vi "TDC_DAQV19_muon.vi"(8 "error in (no error)":errorcluster, 9 "stop":bool=TRUE, 10 "save data":bool=TRUE, 11 "SMA mode":bool=TRUE) -> (3 "rate":dbl)   [LabVIEW 2017]
uses:
  <vilib>/Utility/file.llb/Write Delimited Spreadsheet (DBL).vi
  <vilib>/Utility/file.llb/Write Delimited Spreadsheet (I64).vi
panel:
  out "substring 2":string
  out "error out 3":errorcluster
  out "substring":string
  in  "factor":i32=128
  in  "displayCR":bool=TRUE
  in  "Counter Setting":dbl=100000.0 format="%#_13g"
  in  "replace dat":bool
  in  "append csv":bool=TRUE
  out "concatenated string":string
  out "number":u32=23
  out "element":string
  out "fine":u64=375 format="%x"
  in  "UDP Config":bool=TRUE
  in  "data  path":path=path "G:/tdc/2017"
  out "cal 2":u64[](graph)
  in  "Thresholds (mV)":u16[](array[numeric])=[580, 580, 580, 580, 600, 600, 600, 600, 580, 580, 600, 600, 600, 600, 600, 600, 580, 580, 600, 600, 600, 600, 600, 600, 580, 580, 600, 600, 600, 600, 600, 600]
  out "error out 2":errorcluster={"status"=TRUE, "code"=1, "source"="Dequeue Element in TDC_DAQV18_NewStructure.vi"}
  in  "display":bool=TRUE
  in  "Thresholds":u16=580
  in  "one key for threshold":bool=TRUE
  in  "RST":bool
  in  "通道数量":i32=64
  out "Cal Table":u32[](array[numeric])
  in  "channel for cal":i32
  out "channel number":u64
  in  "bytes to read":i32=320
  out "Calibration Counter":i32=100000
  out "Event index":i32=97959
  out "cal":u32[](graph)
  out "error out":errorcluster
  out "appended path":path=path "G:/tdc/2017/test_20240612_084516.dat"
  in  "filename":string="test"
  in  "Events":i32=110000 min=1
  in  "timeout (ms)":i32=10000
  in  "address":string="192.168.10.23"
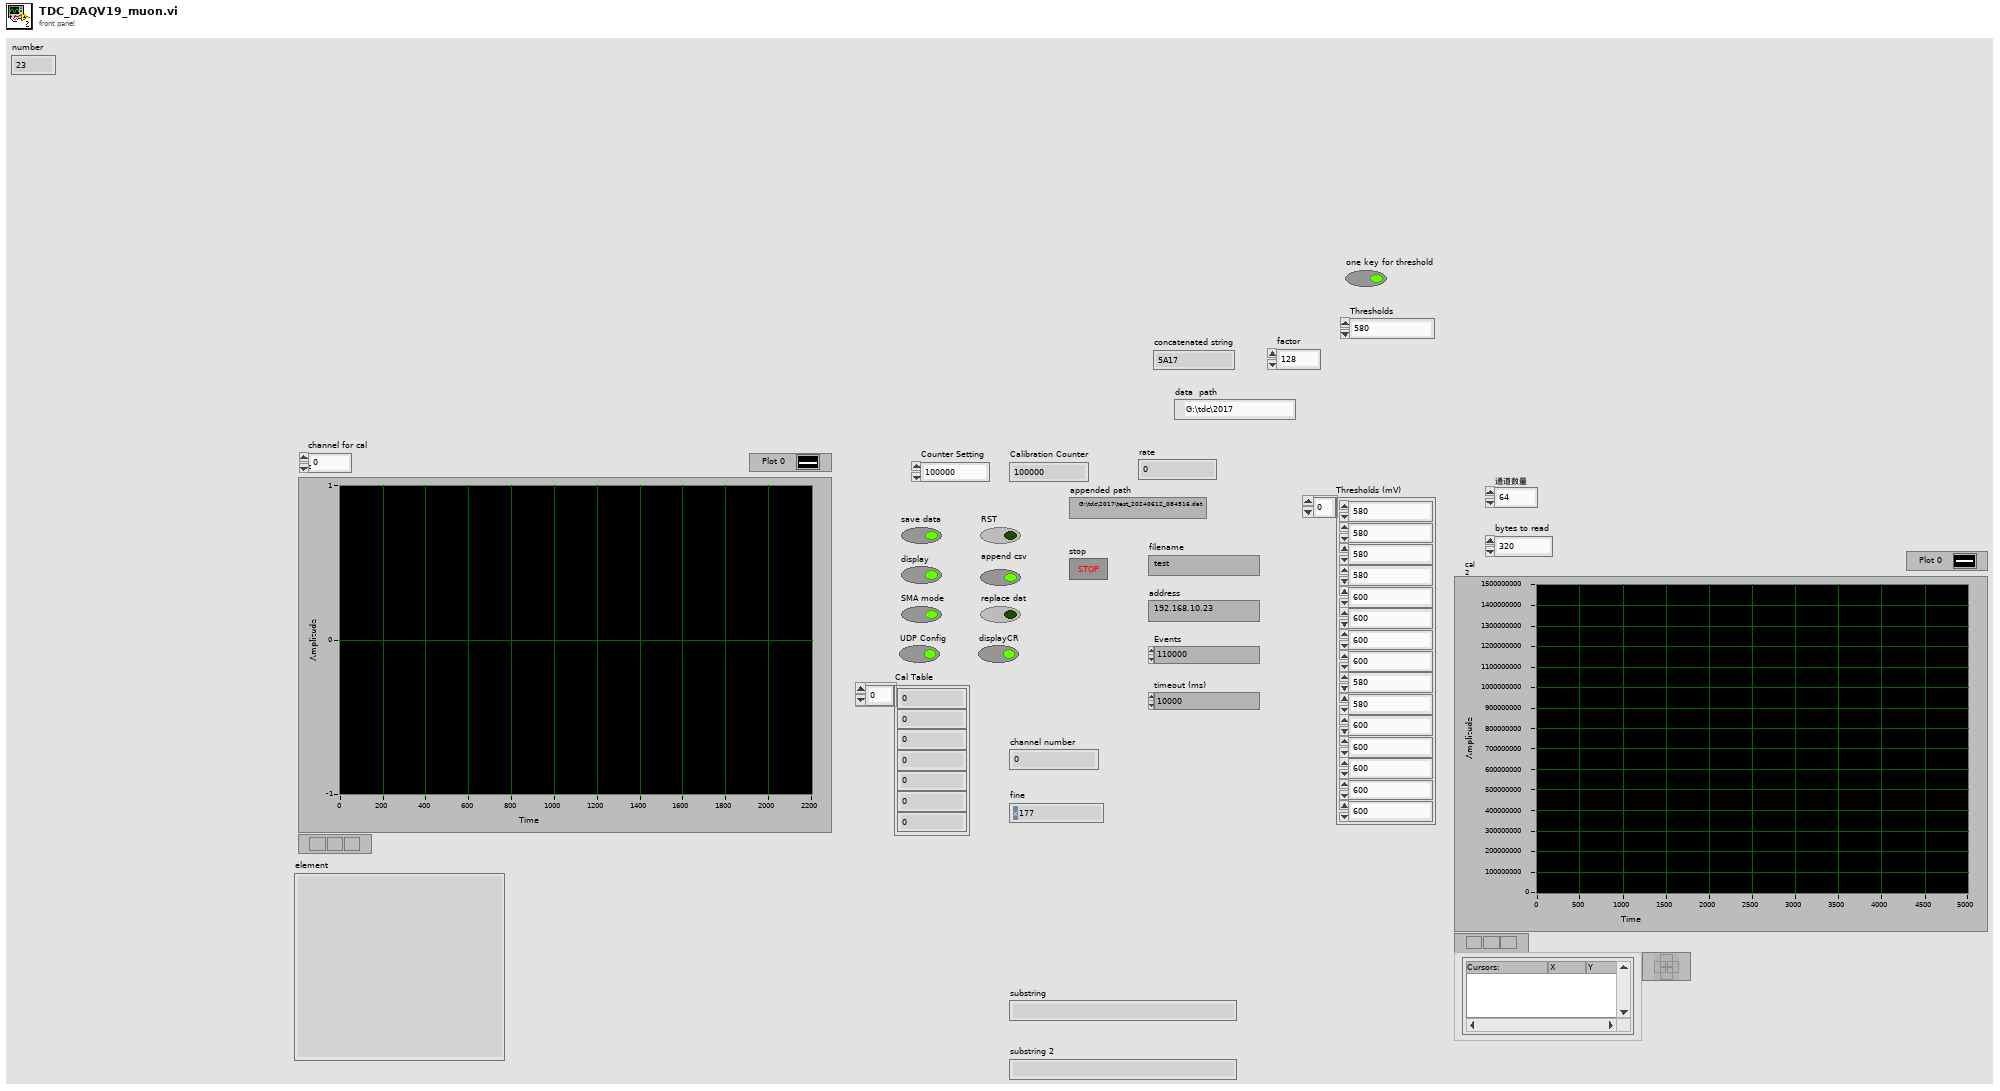
[diagram p1: front panel]
types:
  T1 = enum16{"open", "replace", "create", "open or create", "replace or create", "replace or create with confirmation"}
  T2 = enum16{"Standard", "Buffered", "CRLF", "Immediate"}
  T3 = enum16{"big-endian, network order", "native, host order", "little-endian"}
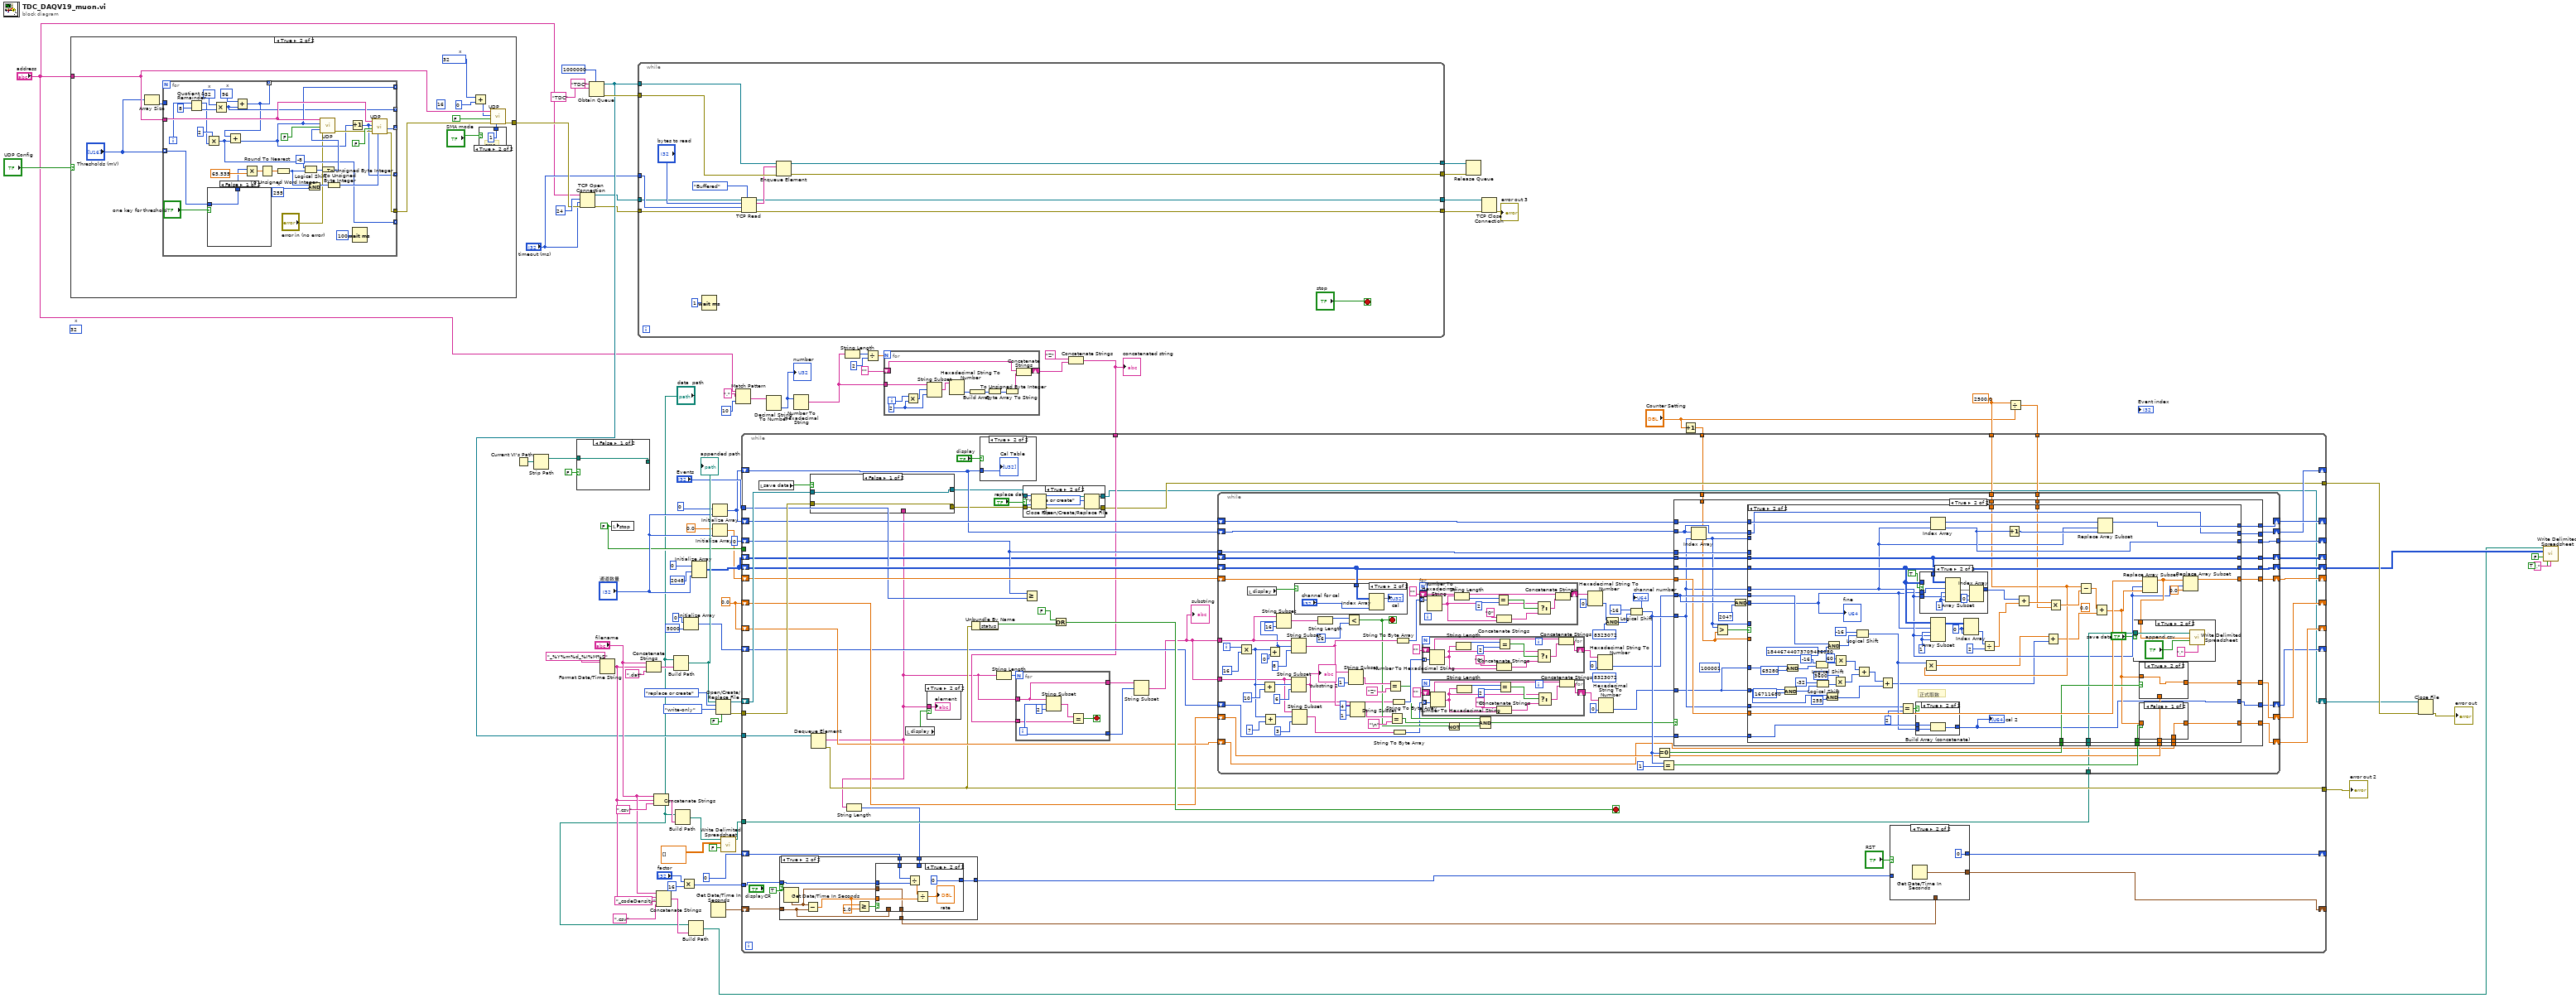
[diagram p0: block diagram]
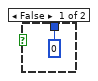
[diagram p3: hidden frame]
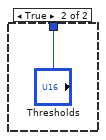
[diagram p4: hidden frame]
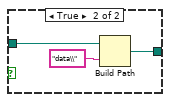
[diagram p5: hidden frame]
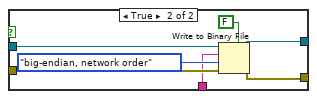
[diagram p7: hidden frame]
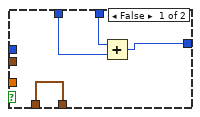
[diagram p10: hidden frame]
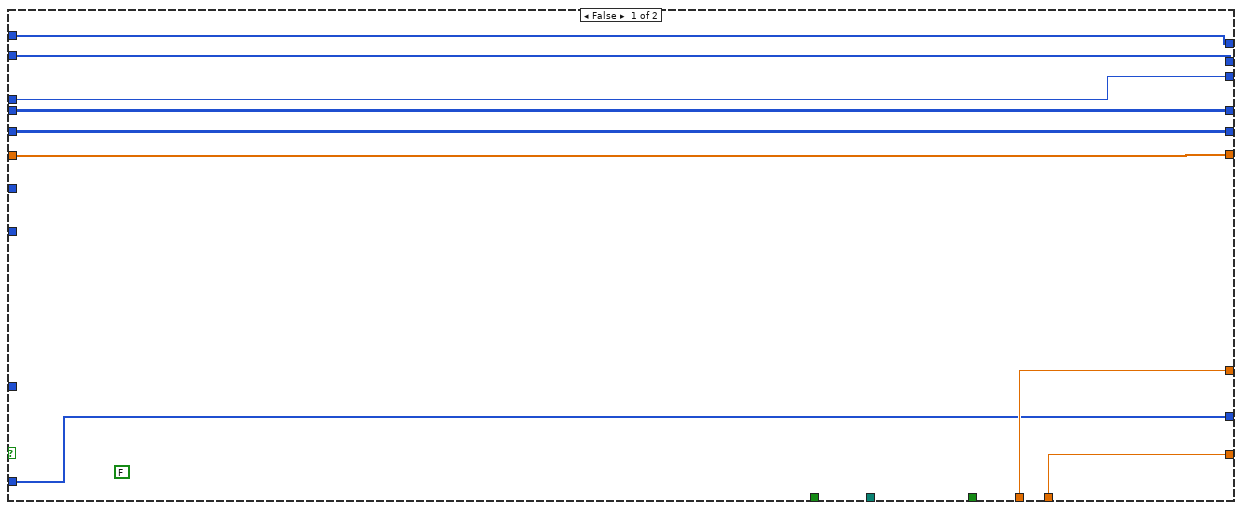
[diagram p14: hidden frame]
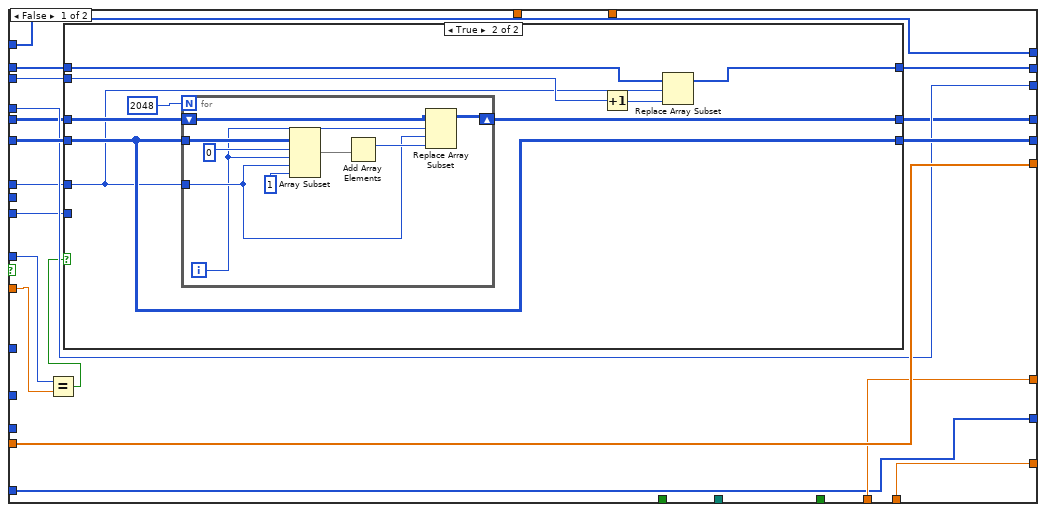
[diagram p15: hidden frame]
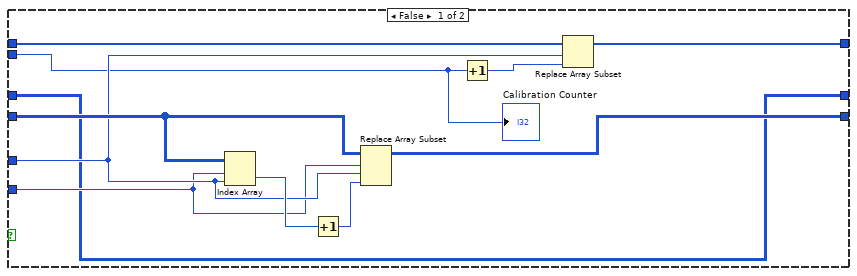
[diagram p16: hidden frame]
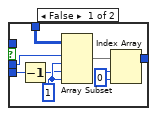
[diagram p19: hidden frame]
diagram:
  w10 = 2500.0 ("x")
  (unwired) u16 32  # x
  w54 = FALSE ("stop")
  w64 = 0.0
  n1 = case shown="True" "UDP Config" {
    tunnel: "address" -> [_ w97]
    tunnel: [_ w94] -> w55
    frame False {
    }
    frame True {
      (unwired) u32 16 ("Address")
      w88 = u16 32  # x
      n2 = Array Size(array="Thresholds (mV)") -> (size(s)=w91:i32)
      n3 = for {
        tunnel: w97 -> [w127]
        tunnel: "Thresholds (mV)" -> [w113] mode=indexing
        tunnel: [w121] -> _ mode=indexing
        tunnel: [w116] -> w95
        tunnel: w91 -> [_]
        tunnel: [w107] -> _ mode=indexing
        tunnel: [w106] -> _ mode=indexing
        tunnel: [w105] -> _ mode=indexing
        tunnel: [w104] -> _ mode=indexing
        tunnel: [w103] -> _ mode=indexing
        i -> [w108]
        w109 = u16 96  # x
        w110 = u16 32  # x
        w123 = u16 255  # x
        n4 = Quotient & Remainder(x=w108, y=8) -> (x-y*floor(x/y)=w102:i32, floor(x/y)=w111:i32)
        n5 = Multiply(x=2, y=w102) -> (x*y=w103:i32)
        n6 = case shown="False" "one key for threshold" {
          tunnel: [w133 "Thresholds"] -> w114
          tunnel: w113 -> [w133 _]
          frame False {
          }
          frame True {
          }
        }
        n7 = Multiply(x=w110, y=w111) -> (x*y=w105:i32)
        n8 = Add(x=w109, y=w105) -> (x+y=w104:i32)
        n9 = Add(x=w104, y=w103) -> (x+y=w107:i32)
        n10 = Multiply(x=w114, y=65.535) -> (x*y=w130:dbl)
        n11 = Round To Nearest(number=w130) -> (nearest integer value=w128:dbl)
        n12 = To Unsigned Word Integer(number=w128) -> (unsigned 16bit integer=w118:u16)
        n13 = Logical Shift(y=i16 -8, x=w118) -> (x << y=w125:u16)
        n14 = And(x=w118, y=w123) -> (x .and. y?=w122:u16)
        n15 = To Unsigned Byte Integer(number=w125) -> (unsigned 8bit integer=w124:u8)
        n16 = call "UDP.vi"("In"=w124, "error in (no error)"="error in (no error)", "Read (TRUE)"=FALSE, "Address"=w107, "IP address"=w127) -> ("error out"=w117:errorcluster)  [unwired: 4 in, 1 out]
        n17 = To Unsigned Byte Integer(number=w122) -> (unsigned 8bit integer=w120:u8)
        n18 = Increment(x=w107) -> (x+1=w106:i32)
        n19 = Wait (ms)(milliseconds to wait=u32 100) -> ()  [unwired: 1 out]
        n20 = call "UDP.vi"("In"=w120, "error in (no error)"=w117, "Read (TRUE)"=FALSE, "Address"=w106, "IP address"=w127) -> ("error out"=w116:errorcluster, "Out"=w121:u8)  [unwired: 4 in]
      }
      n21 = Add(x=w88, y=u32 0 ("Address")) -> (x+y=w87:u32)
      n22 = case shown="True" "SMA mode" {
        tunnel: [u8 0 ("In") u8 1 ("In")] -> w93
        frame False {
        }
        frame True {
          # "sma"
        }
      }
      n23 = call "UDP.vi"("In"=w93, "error in (no error)"=w95, "Read (TRUE)"=FALSE, "Address"=w87, "IP address"=w97) -> ("error out"=w94:errorcluster)  [unwired: 4 in, 1 out]
    }
  }
  n24 = Current VI's Path() -> (path=w80:path)
  n25 = Strip Path(path=w80) -> (stripped path=w79:path)  [unwired: 1 out]
  n26 = case shown="False" FALSE {
    tunnel: w79 -> [w135 w137]
    tunnel: [w135 w136] -> _
    frame False {
    }
    frame True {
      n27 = Build Path(base path=w137, name or relative path="data\\") -> (appended path=w136:path)
    }
  }
  n28 = TCP Open Connection(address="address", remote port or service name=u16 24 ("port"), timeout ms (60000)="timeout (ms)", error in (no error)=w55) -> (connection ID=w38:refnum<k5>, error out=w39:errorcluster)  [unwired: 1 in]
  n29 = Obtain Queue(max queue size (-1, unlimited)=1000000, name (unnamed)="TDC", element data type="TDC" ("name (unnamed)")) -> (queue out=w40:refnum<queue>, error out=w41:errorcluster)  [unwired: 2 in, 1 out]
  n30 = Format Date/Time String(time format string (%c)="_%Y%m%d_%I%M%S") -> (date/time string=w52:string)  [unwired: 2 in]
  n31 = local write "stop"(w54) -> ()
  n32 = while {
    tunnel: w40 -> [w152]
    tunnel: w41 -> [w151]
    tunnel: w39 -> [w149]
    tunnel: "timeout (ms)" -> [w148]
    tunnel: w38 -> [w147]
    tunnel: [w145] -> w37
    tunnel: [w144] -> w36
    tunnel: [w142] -> w35
    tunnel: [w141] -> w34
    stop <- "stop" stop-if-true
    n33 = Wait (ms)(milliseconds to wait=u32 1) -> ()  [unwired: 1 out]
    n34 = TCP Read(connection ID=w147, bytes to read="bytes to read", error in (no error)=w149, 7:T2."Buffered" ("mode (standard)"), 9:w148) -> (connection ID out=w145:refnum<k5>, data out=w146:string, error out=w144:errorcluster)
    n35 = Enqueue Element(queue=w152, element=w146, error in (no error)=w151) -> (queue out=w142:refnum<queue>, error out=w141:errorcluster)  [unwired: 1 in, 1 out]
  }
  n36 = Concatenate Strings("filename", w52, ".dat") -> (w78:string)
  n37 = Concatenate Strings("filename", w52, ".csv") -> (w66:string)
  n38 = Concatenate Strings("filename", w52, "_codeDensity" ("string"), ".csv") -> (w49:string)
  n39 = Build Path(base path="data  path", name or relative path=w78) -> (appended path=w77:path)
  "appended path" <- w77
  n40 = Build Path(base path="data  path", name or relative path=w66) -> (appended path=w61:path)
  n41 = Multiply(x="factor", y=16) -> (x*y=w3:i32)
  n42 = Initialize Array(u32 0 ("element"), 5000 ("dimension size")) -> (w28:u32[])
  n43 = Build Path(base path="data  path", name or relative path=w49) -> (appended path=w46:path)
  n44 = Initialize Array(u32 0 ("element"), 2048 ("dimension size"), "通道数量") -> (w63:u32[][])
  n45 = Get Date/Time In Seconds() -> (seconds since 1Jan1904=w56:timestamp)
  n46 = Initialize Array(u32 0 ("element"), "通道数量") -> (w65:u32[])
  n47 = Initialize Array(0.0, "通道数量") -> (w30:dbl[])
  n48 = Open/Create/Replace File(file path (use dialog)=w77, operation (0:open)=T1."replace or create", access (0:read/write)=enum16{"read/write", "read-only", "write-only"}."write-only", disable buffering (F)=FALSE) -> (refnum out=w82:refnum<file>, error out=w81:errorcluster)  [unwired: 2 in, 1 out]
  n49 = call-poly <vilib>:"Write Delimited Spreadsheet.vi"("file path (dialog if empty)"=w61, "2D data"=dbl[][] [], "append to file? (new file:F)"=FALSE) -> ("new file path (Not A Path if cancelled)"=w60:path)  [unwired: 11 in, 1 out]
  n50 = Match Pattern(string="address", regular expression="." ("search string"), offset (0)=10) -> (after substring=w17:string)  [unwired: 3 out]
  n51 = Decimal String To Number(string=w17) -> (number=w16:i32)  [unwired: 2 in, 1 out]
  "number" <- w16
  n52 = Number To Hexadecimal String(2:w16) -> (0:w14:string)  [unwired: 1 in]
  n53 = String Length(string=w14) -> (length=w22:i32)
  n54 = Divide(x=w22, y=2) -> (x/y=w23:dbl)
  n55 = for {
    N: w23 -> [_]
    shift-right: [w163] -> w13
    shift-left: "" ("format string") -> [w162]
    tunnel: w14 -> [w153]
    i -> [w161]
    w155 = 2 ("y")
    n56 = Multiply(x=w161, y=w155) -> (x*y=w154:i32)
    n57 = String Subset(string=w153, offset (0)=w154, length (rest)=w155) -> (substring=w156:string)
    n58 = Hexadecimal String To Number(string=w156) -> (number=w160:u32)  [unwired: 2 in, 1 out]
    n59 = Build Array(w160) -> (w159:u32[])
    n60 = To Unsigned Byte Integer(number=w159) -> (unsigned 8bit integer=w158:u8[])
    n61 = Byte Array To String(unsigned byte array=w158) -> (string=w157:string)
    n62 = Concatenate Strings(w162, w157) -> (w163:string)
  }
  n63 = Concatenate Strings("Z", w13) -> (w12:string)
  "concatenated string" <- w12
  n64 = Release Queue(queue=w35, error in (no error)=w34) -> ()  [unwired: 1 in, 3 out]
  n65 = TCP Close Connection(connection ID=w37, error in (no error)=w36) -> (error out=→"error out 3":errorcluster)  [unwired: 1 in, 1 out]
  n66 = Increment(x="Counter Setting") -> (x+1=w6:dbl)
  n67 = Divide(x=w10, y="Counter Setting") -> (x/y=w9:dbl)
  n68 = while {
    tunnel: w81 -> [w217]
    tunnel: [w191] -> w33
    tunnel: [w175] -> w74
    shift-right: [w214] -> w47
    shift-left: w63 -> [w215]
    shift-right: [w200] -> _
    shift-left: w30 -> [w213]
    tunnel: "Events" -> [w211]
    shift-right: [w210] -> _
    shift-left: w65 -> [w209]
    shift-right: [w208] -> _
    shift-left: u32 0 ("element") -> [w207]
    shift-right: [w206] -> _
    shift-left: w65 -> [w193]
    shift-right: [w205] -> _
    shift-left: w64 -> [w202]
    shift-right: [w204] -> _
    shift-left: w64 -> [w203]
    shift-right: [w195] -> _
    shift-left: w63 -> [w201]
    tunnel: w60 -> [w187]
    shift-right: [w199] -> _
    shift-left: 0 -> [w169]
    shift-right: [w197] -> _
    shift-left: w56 -> [w196]
    tunnel: w54 -> [_]
    tunnel: w40 -> [w192]
    shift-right: [w188] -> _
    shift-left: w28 -> [w189]
    tunnel: w12 -> [w183]
    tunnel: w10 -> [w181]
    tunnel: w9 -> [w180]
    shift-right: [w174] -> w8
    shift-left: w82 -> [w216]
    tunnel: w6 -> [w173]
    tunnel: w3 -> [w166]
    stop <- w212 stop-if-true
    n69 = local read "save data"() -> (w168:bool)
    n70 = Dequeue Element(queue=w192) -> (element=w179:string, error out=w191:errorcluster)  [unwired: 2 in, 2 out]
    n71 = case shown="False" w168 {
      tunnel: w217 -> [w219 w227]
      tunnel: w216 -> [w220 w226]
      tunnel: w179 -> [_ w223]
      tunnel: [w220 w222] -> w178
      tunnel: [w219 w221] -> w176
      frame False {
      }
      frame True {
        n72 = Write to Binary File(file (use dialog)=w226, data=w223, error in=w227, 5:FALSE ("prepend array or string size? (T)"), 9:T3."big-endian, network order" ("byte order (0:big-endian, network order)")) -> (refnum out=w222:refnum<file>, error out=w221:errorcluster)  [unwired: 1 in, 1 out]
      }
    }
    n73 = String Length(string=w179) -> (length=w170:i32)
    n74 = case shown="True" TRUE {
      tunnel: w196 -> [w244 w249]
      tunnel: [w244 w250] -> w172
      tunnel: w169 -> [w243 w248]
      tunnel: w170 -> [_ w247]
      tunnel: [w243 w246] -> w171
      tunnel: w166 -> [_ w245]
      frame False {
      }
      frame True {
        n75 = Get Date/Time In Seconds() -> (seconds since 1Jan1904=w251:timestamp)
        n76 = Subtract(x=w251, y=w249) -> (x-y=w253:dbl)
        n77 = Greater Or Equal?(x=w253, y=1.0) -> (x >= y?=w254:bool)
        n78 = case shown="True" w254 {
          tunnel: w253 -> [_ w265]
          tunnel: w251 -> [_ w263]
          tunnel: [w258 w263] -> w250
          tunnel: w249 -> [w258 _]
          tunnel: w248 -> [w257 w260]
          tunnel: w247 -> [w256 _]
          tunnel: [w255 0] -> w246
          tunnel: w245 -> [_ w259]
          frame False {
            n79 = Add(x=w256, y=w257) -> (x+y=w255:i32)
          }
          frame True {
            n80 = Divide(x=w260, y=w259) -> (x/y=w262:dbl)
            n81 = Divide(x=w262, y=w265) -> (x/y=→"rate":dbl)
          }
        }
      }
    }
    n82 = local read "display"() -> (w167:bool)
    n83 = case shown="True" w167 {
      tunnel: w179 -> [_ w218]
      frame False {
      }
      frame True {
        "element" <- w218
      }
    }
    n84 = Unbundle By Name(w191) -> ("status"=w190:bool)
    n85 = case shown="True" "display" {
      tunnel: w193 -> [_ w266]
      frame False {
      }
      frame True {
        "Cal Table" <- w266
      }
    }
    n86 = String Length(string=w179) -> (length=w186:i32)
    n87 = for {
      N: w186 -> [_]
      tunnel: w179 -> [w239]
      tunnel: [w239] -> w185
      tunnel: [w238] -> w184
      tunnel: w183 -> [w237]
      i -> [w238]
      stop <- w240 stop-if-true
      n88 = String Subset(string=w239, offset (0)=w238, length (rest)=2 ("length (rest)")) -> (substring=w241:string)
      n89 = Equal?(x=w241, y=w237) -> (x = y?=w240:bool)
    }
    n90 = case shown="True" "replace dat" {
      tunnel: w178 -> [w229 w235]
      tunnel: [w229 w234] -> w174
      tunnel: w176 -> [w228 w231]
      tunnel: [w228 w230] -> w175
      frame False {
      }
      frame True {
        n91 = Close File(refnum=w235, error in=w231) -> (path=w236:path, error out=w232:errorcluster)
        n92 = Open/Create/Replace File(file path (use dialog)=w236, error in=w232, operation (0:open)=T1."replace or create") -> (refnum out=w234:refnum<file>, error out=w230:errorcluster)  [unwired: 3 in, 1 out]
      }
    }
    n93 = Greater Or Equal?(x=w207, y=w211) -> ()  [unwired: 1 out]
    n94 = Or(x=FALSE, y=w190) -> (x .or. y?=w212:bool)
    n95 = String Subset(string=w185, offset (0)=w184) -> (substring=w164:string)  [unwired: 1 in]
    "substring" <- w164
    n96 = while {
      tunnel: w164 -> [w291]
      shift-right: [w344] -> w214
      shift-left: w215 -> [w342]
      shift-right: [w340] -> w200
      shift-left: w213 -> [w341]
      shift-right: [w335] -> w210
      shift-left: w209 -> [w334]
      tunnel: [w333] -> w208
      tunnel: w207 -> [w332]
      shift-right: [w330] -> w206
      shift-left: w193 -> [w331]
      shift-right: [w325] -> w205
      shift-left: w202 -> [w323]
      shift-right: [w321] -> w204
      shift-left: w203 -> [w322]
      tunnel: w187 -> [w320]
      shift-right: [w319] -> w195
      shift-left: w201 -> [w285]
      shift-right: [w316] -> w188
      shift-left: w189 -> [w317]
      tunnel: w164 -> [w277]
      tunnel: w181 -> [w293]
      tunnel: w180 -> [w292]
      tunnel: w173 -> [w284]
      i -> [w345]
      stop <- w287 stop-if-true
      (unwired) u64 8323072 ("port")
      n97 = Multiply(x=w345, y=16 ("length (rest)")) -> (x*y=w278:i32)
      n98 = local read "display"() -> (w318:bool)
      n99 = Add(x=w278, y=10 ("length (rest)")) -> (x+y=w308:i32)
      n100 = Add(x=w278, y=7 ("length (rest)")) -> (x+y=w280:i32)
      n101 = Add(x=w278, y=0 ("length (rest)")) -> (x+y=w290:i32)
      n102 = String Subset(string=w291, offset (0)=w290, length (rest)=16 ("y")) -> (substring=w288:string)
      n103 = String Subset(string=w291, offset (0)=w290, length (rest)=8 ("length (rest)")) -> (substring=w294:string)
      n104 = String Subset(string=w277, offset (0)=w308, length (rest)=6 ("length (rest)")) -> (substring=w283:string)
      "substring 2" <- w283
      n105 = String Subset(string=w277, offset (0)=w280, length (rest)=3 ("length (rest)")) -> (substring=w273:string)
      n106 = case shown="True" w318 {
        tunnel: w342 -> [_ w371]
        frame False {
        }
        frame True {
          n107 = Index Array(array=w371, index (col)="channel for cal") -> (element=→"cal":u32[])  [unwired: 1 in]
        }
      }
      n108 = String Length(string=w288) -> (length=w339:i32)
      n109 = Less?(x=w339, y=16) -> (x < y?=w287:bool)
      n110 = String Subset(string=w294, length (rest)=1 ("length (rest)")) -> (substring=w313:string)  [unwired: 1 in]
      n111 = String Subset(string=w294, offset (0)=4, length (rest)=1 ("length (rest)")) -> (substring=w295:string)
      n112 = Equal?(x=w313, y="Z" ("format string")) -> (x = y?=w297:bool)
      n113 = Equal?(x=w295, y="\n" ("format string")) -> (x = y?=w296:bool)
      n114 = String To Byte Array(string=w283) -> (unsigned byte array=w305:u8[])
      n115 = String To Byte Array(string=w273) -> (unsigned byte array=w272:u8[])
      n116 = String To Byte Array(string=w294) -> (unsigned byte array=w347:u8[])
      n117 = for {
        shift-right: [w559] -> w302
        shift-left: "" ("format string") -> [w556]
        tunnel: w347 -> [w560] mode=indexing
        n118 = Number To Hexadecimal String(2:w560) -> (0:w552:string)  [unwired: 1 in]
        n119 = String Length(string=w552) -> (length=w558:i32)
        n120 = Equal?(x=w558, y=2) -> (x = y?=w555:bool)
        n121 = Concatenate Strings("0" ("format string"), w552) -> (w554:string)
        n122 = Select(t=w552, s=w555, f=w554) -> (s? t:f=w551:string)
        n123 = Concatenate Strings(w556, w551) -> (w559:string)
      }
      n124 = for {
        shift-right: [w367] -> w303
        shift-left: "" ("format string") -> [w359]
        tunnel: w305 -> [w368] mode=indexing
        n125 = Number To Hexadecimal String(2:w368) -> (0:w361:string)  [unwired: 1 in]
        n126 = String Length(string=w361) -> (length=w366:i32)
        n127 = Concatenate Strings("0" ("format string"), w361) -> (w363:string)
        n128 = Equal?(x=w366, y=2) -> (x = y?=w364:bool)
        n129 = Select(t=w361, s=w364, f=w363) -> (s? t:f=w360:string)
        n130 = Concatenate Strings(w359, w360) -> (w367:string)
      }
      n131 = for {
        shift-right: [w357] -> w276
        shift-left: "" ("format string") -> [w349]
        tunnel: w272 -> [w358] mode=indexing
        n132 = Number To Hexadecimal String(2:w358) -> (0:w351:string)  [unwired: 1 in]
        n133 = String Length(string=w351) -> (length=w356:i32)
        n134 = Concatenate Strings("0" ("format string"), w351) -> (w353:string)
        n135 = Equal?(x=w356, y=2) -> (x = y?=w354:bool)
        n136 = Select(t=w351, s=w354, f=w353) -> (s? t:f=w350:string)
        n137 = Concatenate Strings(w349, w350) -> (w357:string)
      }
      n138 = Not(x=w287) -> (.not. x?=w286:bool)
      n139 = Compound Arithmetic op=AND(w297, w296, w286) -> (w311:bool)
      n140 = Hexadecimal String To Number(string=w302, default (0uL)=u64 0 ("default (0 U32)")) -> (number=w343:u64)  [unwired: 1 in, 1 out]
      n141 = Hexadecimal String To Number(string=w303, default (0uL)=u64 0 ("default (0 U32)")) -> (number=w301:u64)  [unwired: 1 in, 1 out]
      n142 = Hexadecimal String To Number(string=w276, default (0uL)=u64 0 ("default (0 U32)")) -> (number=w271:u64)  [unwired: 1 in, 1 out]
      n143 = And(x=w343, y=u64 8323072 ("port")) -> (x .and. y?=w336:u64)
      n144 = Logical Shift(y=i16 -16, x=w336) -> (x << y=w328:u64)
      "channel number" <- w328
      n145 = Equal To 0?(x=w328) -> (x = 0?=w326:bool)
      n146 = Equal?(x=w328, y=u64 1) -> (x = y?=w324:bool)
      n147 = case shown="True" w311 {
        tunnel: w301 -> [_ w411]
        tunnel: w332 -> [w377 w401]
        tunnel: w342 -> [w380 w410]
        tunnel: [w380 w409] -> w344
        tunnel: [w379 w406] -> w340
        tunnel: w341 -> [w379 w405]
        tunnel: w328 -> [_ w385]
        tunnel: w334 -> [w378 w404]
        tunnel: [w378 w403] -> w335
        tunnel: [w377 w402] -> w333
        tunnel: w331 -> [w376 w400]
        tunnel: [w376 w399] -> w330
        tunnel: w326 -> [_ w398]
        tunnel: w323 -> [w375 w397]
        tunnel: [w375 w396] -> w325
        tunnel: w324 -> [_ w395]
        tunnel: w322 -> [w374 w394]
        tunnel: [w374 w393] -> w321
        tunnel: w285 -> [w373 w391]
        tunnel: [w373 w390] -> w319
        tunnel: w320 -> [_ w389]
        tunnel: w317 -> [w372 w387]
        tunnel: [w372 w386] -> w316
        tunnel: w293 -> [_ w384]
        tunnel: w292 -> [_ w383]
        tunnel: w284 -> [_ w382]
        tunnel: w271 -> [_ w381]
        frame False {
          (unwired) FALSE
        }
        frame True {
          (unwired) 100001 ("y")
          n148 = Index Array(array=w400, index=w385) -> (element=w392:u32)
          n149 = Greater?(x=w392, y=w382) -> (0:w388:bool)
          n150 = And(x=w411, y=u64 2047 ("port")) -> (x .and. y?=w407:u64)
          n151 = case shown="True" w388 {
            tunnel: w411 -> [_ w523]
            tunnel: w410 -> [w429 w509]
            tunnel: [w428 w509] -> w409
            tunnel: w407 -> [w420 w482]
            tunnel: [w427 w493] -> w406
            tunnel: w405 -> [w427 w516]
            tunnel: w401 -> [w425 _]
            tunnel: w385 -> [w423 w491]
            tunnel: w404 -> [w426 w515]
            tunnel: [w426 w514] -> w403
            tunnel: [w425 w512] -> w402
            tunnel: w392 -> [w421 _]
            tunnel: w400 -> [w424 w511]
            tunnel: [w422 w511] -> w399
            tunnel: w398 -> [_ w504]
            tunnel: w397 -> [w419 w503]
            tunnel: [w419 w502] -> w396
            tunnel: w395 -> [_ w501]
            tunnel: w394 -> [w418 w500]
            tunnel: [w418 w499] -> w393
            tunnel: w392 -> [w416 _]
            tunnel: w382 -> [w413 _]
            tunnel: w391 -> [w415 w495]
            tunnel: [w414 w495] -> w390
            tunnel: w389 -> [_ w494]
            tunnel: w387 -> [w412 w488]
            tunnel: [w412 w486] -> w386
            tunnel: w385 -> [_ w483]
            tunnel: w384 -> [_ w480]
            tunnel: w383 -> [_ w481]
            tunnel: w381 -> [_ w475]
            tunnel: w381 -> [_ w463]
            frame False {
              n152 = Equal?(x=w416, y=w413) -> (x = y?=w417:bool)
              n153 = case shown="True" w417 {
                tunnel: w429 -> [w440 w446]
                tunnel: [w438 w446] -> w428
                tunnel: w424 -> [w436 w444]
                tunnel: w423 -> [w435 w441]
                tunnel: [w433 w443] -> w422
                tunnel: w421 -> [w432 w442]
                tunnel: w420 -> [w431 _]
                tunnel: w415 -> [w430 w448]
                tunnel: [w430 w447] -> w414
                frame False {
                  n154 = Index Array(array=w440, index (row)=w431, index (col)=w435) -> (element=w439:u32)
                  n155 = Increment(x=w439) -> (x+1=w437:u32)
                  n156 = Replace Array Subset(array=w440, new element=w437, index (row)=w431, index (col)=w435) -> (w438:u32[][])
                  n157 = Increment(x=w432) -> (x+1=w434:u32)
                  n158 = Replace Array Subset(array=w436, new element=w434, index=w435) -> (w433:u32[])
                  "Calibration Counter" <- w432
                }
                frame True {
                  n159 = for {
                    N: 2048 -> [_]
                    tunnel: w446 -> [w458]
                    tunnel: w441 -> [w451]
                    shift-right: [w453] -> w447
                    shift-left: w448 -> [w454]
                    i -> [w450]
                    n160 = Array Subset(array=w458, index (row)=0 ("索引"), length (row)=w450, index (col)=w451, length (col)=1 ("长度")) -> (w455:u32[][])
                    n161 = Add Array Elements(numeric array=w455) -> (sum=w452:u32)
                    n162 = Replace Array Subset(array=w454, new element=w452, index (row)=w450, index (col)=w451) -> (w453:u32[][])
                  }
                  n163 = Increment(x=w442) -> (x+1=w445:u32)
                  n164 = Replace Array Subset(array=w444, new element=w445, index=w441) -> (w443:u32[])
                }
              }
            }
            frame True {
              (unwired) 0.0 ("x")
              w506 = 0 ("索引 (行)")
              w508 = 1 ("长度")
              # "正式取数"
              n165 = And(x=w463, y=u64 16711680 ("port")) -> (x .and. y?=w472:u64)
              n166 = And(x=w475, y=u64 65280 ("port")) -> (x .and. y?=w478:u64)
              n167 = Logical Shift(y=i16 -16, x=w478) -> (x << y=w469:u64)
              n168 = Logical Shift(y=i16 -32, x=w472) -> (x << y=w471:u64)
              n169 = And(x=w463, y=u64 255 ("port")) -> (x .and. y?=w462:u64)
              n170 = And(x=w523, y=u64 18446744073709486080 ("port")) -> (x .and. y?=w520:u64)
              n171 = Multiply(x=u64 3600, y=w471) -> (x*y=w466:u64)
              n172 = Multiply(x=u64 60, y=w469) -> (x*y=w467:u64)
              n173 = Logical Shift(y=i16 -16, x=w520) -> (x << y=w487:u64)
              n174 = Add(x=w467, y=w466) -> (x+y=w465:u64)
              n175 = Add(x=w465, y=w462) -> (x+y=w459:u64)
              n176 = Equal?(x=w483, y=u32 2) -> (x = y?=w485:bool)
              n177 = case shown="True" w485 {
                tunnel: w488 -> [w524 w527]
                tunnel: w487 -> [_ w526]
                tunnel: [w524 w525] -> w486
                frame False {
                }
                frame True {
                  n178 = Build Array (concatenate)(w527, w526) -> (w525:u64[])
                }
              }
              "cal 2" <- w486
              n179 = case shown="True" TRUE {
                tunnel: [w534 w542] -> w518
                tunnel: w509 -> [_ _]
                tunnel: w491 -> [w539 w540]
                tunnel: w482 -> [w537 w545]
                tunnel: w495 -> [w538 w546]
                frame False {
                  w533 = 0 ("index (row)")
                  w536 = 1 ("长度")
                  n180 = Decrement(x=w539) -> (x-1=w532:u64)
                  n181 = Array Subset(array=w538, index (row)=w537, length (row)=w536, index (col)=w532, length (col)=w536) -> (w535:u32[][])
                  n182 = Index Array(array=w535, index (row)=w533, index (col)=w533) -> (element=w534:u32)
                }
                frame True {
                  w541 = 0 ("index (row)")
                  w544 = 1 ("长度")
                  n183 = Array Subset(array=w546, index (row)=w545, length (row)=w544, index (col)=w540, length (col)=w544) -> (w543:u32[][])
                  n184 = Index Array(array=w543, index (row)=w541, index (col)=w541) -> (element=w542:u32)
                }
              }
              n185 = Multiply(x=w487, y=w480) -> (x*y=w461:dbl)
              n186 = Index Array(array=w515, index=w491) -> (element=w512:u32)
              n187 = Array Subset(array=w509, index (row)=w482, length (row)=w508, index (col)=w491, length (col)=w508) -> (w507:u32[][])
              n188 = Index Array(array=w507, index (row)=w506, index (col)=w506) -> (element=w505:u32)
              n189 = Divide(x=w505, y=u32 2) -> (x/y=w510:dbl)
              n190 = Increment(x=w512) -> (x+1=w513:u32)
              n191 = Add(x=w518, y=w510) -> (x+y=w517:dbl)
              n192 = Add(x=w461, y=w459) -> (x+y=w460:dbl)
              n193 = Multiply(x=w517, y=w481) -> (x*y=w497:dbl)
              n194 = Subtract(x=w480, y=w497) -> (x-y=w479:dbl)
              n195 = Add(x=w479, y=w460) -> (x+y=w498:dbl)
              n196 = Replace Array Subset(array=w515, new element=w513, index=w491) -> (w514:u32[])
              n197 = case shown="True" w504 {
                tunnel: w498 -> [_ w550]
                tunnel: [w549 w550] -> w502
                tunnel: w503 -> [w549 _]
                frame False {
                }
                frame True {
                }
              }
              n198 = case shown="False" w501 {
                tunnel: [w547 w548] -> w499
                tunnel: w500 -> [w547 _]
                tunnel: w498 -> [_ w548]
                frame False {
                }
                frame True {
                }
              }
              n199 = Replace Array Subset(array=w516, new element=w498, index=w491) -> (w492:dbl[])
              n200 = case shown="True" "save data" {
                tunnel: w494 -> [_ w531]
                tunnel: w492 -> [_ w529]
                frame False {
                }
                frame True {
                  n201 = call-poly <vilib>:"Write Delimited Spreadsheet.vi"("file path (dialog if empty)"=w531, "1D data"=w529, "append to file? (new file:F)"="append csv", "delimiter (\\t)"="," ("delimiter (\\t)")) -> ()  [unwired: 10 in, 2 out]
                }
              }
              n202 = Replace Array Subset(array=w492, new element=0.0 ("new element/subarray"), index=w491) -> (w493:dbl[])
              "fine" <- w482
            }
          }
        }
      }
    }
    n203 = case shown="True" "RST" {
      tunnel: w171 -> [w268 _]
      tunnel: [w268 0] -> w199
      tunnel: [w267 w269] -> w197
      tunnel: w172 -> [w267 _]
      frame False {
      }
      frame True {
        n204 = Get Date/Time In Seconds() -> (seconds since 1Jan1904=w269:timestamp)
      }
    }
  }
  "error out 2" <- w33
  n205 = Close File(refnum=w8, error in=w74) -> (error out=→"error out":errorcluster)  [unwired: 1 out]
  n206 = call-poly <vilib>:"Write Delimited Spreadsheet.vi"("file path (dialog if empty)"=w46, "2D data"=w47, "append to file? (new file:F)"=FALSE, "transpose? (no:F)"=TRUE, "delimiter (\\t)"="," ("delimiter (\\t)")) -> ()  [unwired: 9 in, 2 out]
